vi "SetDriveSpeeds.vi"(8 "error in":errorcluster, 10 "Right Value":dbl, 11 "Left Value":dbl) -> (0 "error out":errorcluster)   [LabVIEW 2016]
uses:
  Robot Global Data.vi
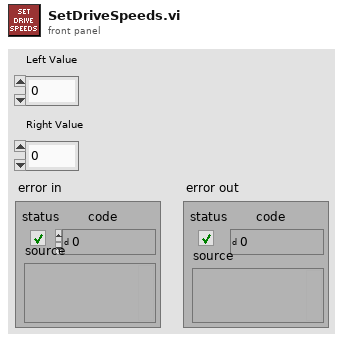
[diagram p1: front panel]
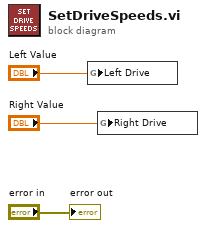
[diagram p0: block diagram]
diagram:
  n1 = global write "Robot Global Data.vi" "Left Drive"("Left Value") -> ()
  n2 = global write "Robot Global Data.vi" "Right Drive"("Right Value") -> ()
  "error out" <- "error in"
